vi "writeUART.vi"(8 "error in (no error)":errorcluster, 10 "write buffer":string, 11 "GiaoTiep in":refnum<class "GiaoTiepUART.lvclass">) -> (0 "error out":errorcluster, 2 "(DataWrite)":string, 3 "GiaoTiep out":refnum<class "GiaoTiepUART.lvclass">)   [LabVIEW 2017, in "LibraryGcode.lvlib" / "GiaoTiepUART.lvclass"]
uses:
  GiaoTiepUART.lvclass
  GiaoTiepUART.lvclass/GiaoTiepUART.ctl
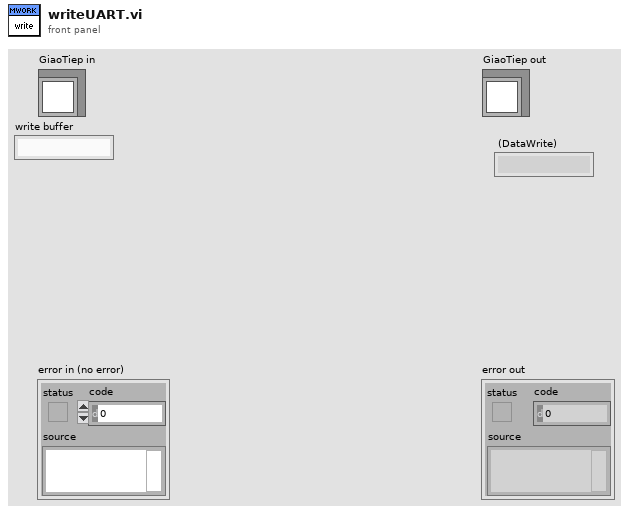
[diagram p1: front panel]
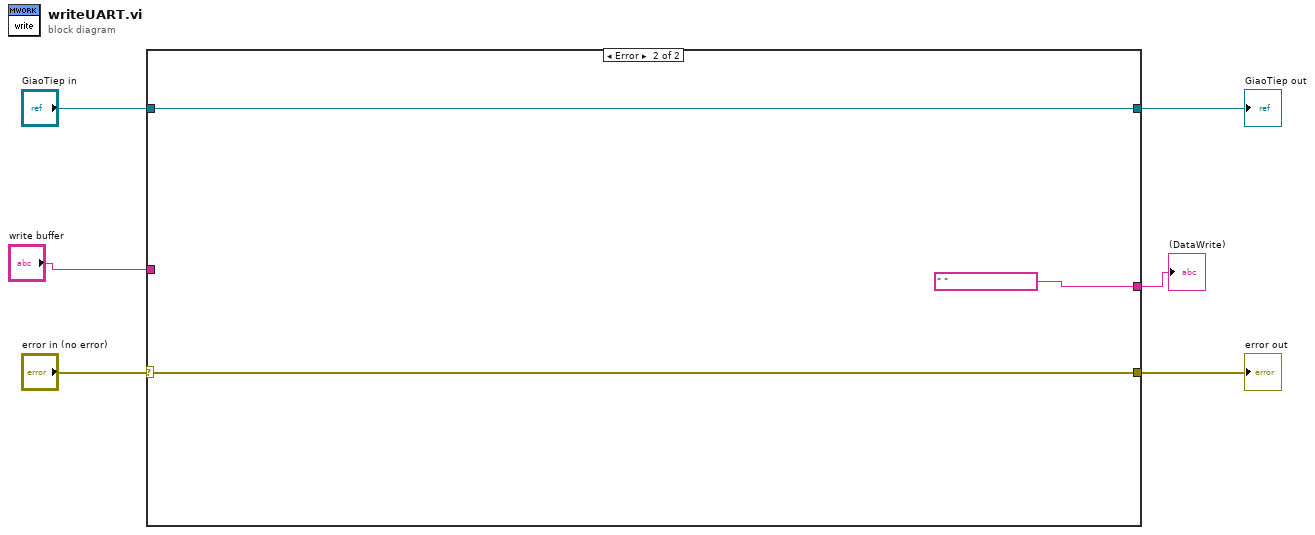
[diagram p0: block diagram]
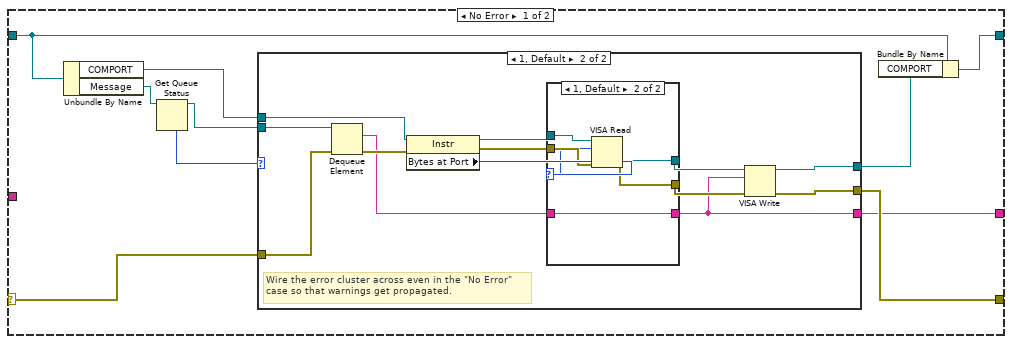
[diagram p2: hidden frame]
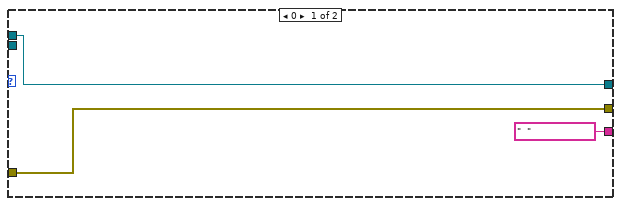
[diagram p3: hidden frame]
diagram:
  n1 = case shown="Error" "error in (no error)" {
    selector: "error in (no error)" -> [w16 w44]
    tunnel: [w15 w44] -> w5
    tunnel: [w13 w43] -> w3
    tunnel: "GiaoTiep in" -> [w12 w43]
    tunnel: "write buffer" -> [_ _]
    tunnel: [w7 " " ("name (unnamed)")] -> w1
    frame No Error {
      n2 = Unbundle By Name(w12) -> ("COMPORT"=w14:refnum<visa-resource-name>, "Message"=w10:refnum<queue>)
      n3 = Get Queue Status(queue=w10) -> (queue out=w8:refnum<queue>, # elements in queue=w9:i32)  [unwired: 2 in, 6 out]
      n4 = case shown="1, Default" w9 {
        tunnel: w16 -> [w18 w24]
        tunnel: [w18 w27] -> w15
        tunnel: w14 -> [w19 w26]
        tunnel: [w19 w25] -> w11
        tunnel: w8 -> [_ w22]
        tunnel: ["  " ("name (unnamed)") w20] -> w7
        frame 0 {
        }
        frame 1, Default {
          # "Wire the error cluster across even in the \"No Error\"\ncase so that warnings get propagated."
          n5 = Dequeue Element(queue=w22, error in (no error)=w24) -> (element=w21:string, error out=w23:errorcluster)  [unwired: 1 in, 2 out]
          n6 = property class="Instr"(reference=w26, error in=w23) -> (reference out=w32:refnum<visa-resource-name>, error out=w31:errorcluster, "Bytes at Port"=w30:u32)
          n7 = case shown="1, Default" w30 {
            selector: w30 -> [_ w37]
            tunnel: w32 -> [w35 w41]
            tunnel: w31 -> [w34 w40]
            tunnel: [w35 w39] -> w29
            tunnel: [w34 w38] -> w28
            tunnel: [w33 w36] -> w20
            tunnel: w21 -> [w33 w36]
            frame 0 {
            }
            frame 1, Default {
              n8 = VISA Read(VISA resource name=w41, byte count=w37, error in (no error)=w40) -> (VISA resource name out=w39:refnum<visa-resource-name>, error out=w38:errorcluster)  [unwired: 2 out]
            }
          }
          n9 = VISA Write(VISA resource name=w29, write buffer=w20, error in (no error)=w28) -> (VISA resource name out=w25:refnum<visa-resource-name>, error out=w27:errorcluster)  [unwired: 1 out]
        }
      }
      n10 = Bundle By Name(cluster=w12, "COMPORT"=w11) -> (w13:refnum<class "GiaoTiepUART.lvclass">)
    }
    frame Error {
    }
  }
  "error out" <- w5
  "GiaoTiep out" <- w3
  "(DataWrite)" <- w1
